vi "Pressure_Honeywell_ADN.vi"() -> (3 "Pressure(kPa)":dbl)   [LabVIEW 2012]
uses:
  <vilib>/Instr/_visa.llb/VISA Configure Serial Port (Instr).vi
panel:
  out "error out":errorcluster
  out "read buffer":string
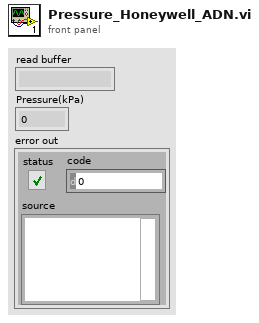
[diagram p1: front panel]
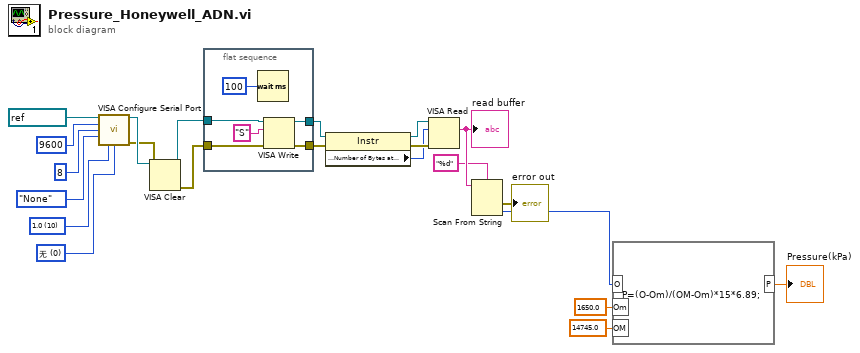
[diagram p0: block diagram]
diagram:
  w18 = u16 0 items=["无", "XON/XOFF", "RTS/CTS", "XON/XOFF & RTS/CTS", "DTR/DSR", "XON/XOFF & DTR/DSR"] ("flow control (0:none)")
  w19 = u16 10 items=["1.0"=10, "1.5"=15, "2.0"=20] ("stop bits (10: 1 bit)")
  n1 = call-poly "VISA Configure Serial Port"("VISA resource name"=refnum<visa-resource-name> "COM18", "baud rate (9600)"=u32 9600, "data bits (8)"=u16 8, "parity (0:none)"=enum16{"None", "Odd", "Even", "Mark", "Space"}."None", "stop bits (10: 1 bit)"=w19, "flow control (0:none)"=w18) -> ("VISA resource name out"=w4:refnum<visa-resource-name>, "error out"=w2:errorcluster)  [unwired: 1 in, 7 out]
  n2 = VISA Clear(VISA resource name=w4, error in (no error)=w2) -> (VISA resource name out=w3:refnum<visa-resource-name>, error out=w1:errorcluster)
  n3 = flat-sequence {
    tunnel: w3 -> [w27]
    tunnel: w1 -> [w26]
    tunnel: [w24] -> w17
    tunnel: [w23] -> w15
    frame #0 {
      n4 = Wait (ms)(milliseconds to wait=u32 100) -> ()  [unwired: 1 out]
      n5 = VISA Write(VISA resource name=w27, write buffer="S", error in (no error)=w26) -> (VISA resource name out=w24:refnum<visa-resource-name>, error out=w23:errorcluster)  [unwired: 1 out]
    }
  }
  n6 = property class="Instr"(reference=w17, error in=w15) -> (reference out=w16:refnum<visa-resource-name>, error out=w14:errorcluster, "Serial Settings:Number of Bytes at Serial Port"=w13:u32)
  n7 = VISA Read(VISA resource name=w16, byte count=w13, error in (no error)=w14) -> (read buffer=w11:string)  [unwired: 3 out]
  "read buffer" <- w11
  n8 = Scan From String(format string="%d", input string=w11) -> (error out=→"error out":errorcluster, output 1=w9:i32)  [unwired: 3 in, 2 out]
  n9 = formula code="P=(O-Om)/(OM-Om)*15*6.89;"("O"=w9, "Om"=1650.0 ("input variable"), "OM"=14745.0 ("input variable")) -> ("P"=→"Pressure(kPa)":dbl)
